vi "Load Machine Configuration.vi"(4 "error in (no error)":errorcluster, 6 "Reload?":bool, 7 "Instance Name":T2) -> (0 "error out":errorcluster, 3 "TC Parameters":T1)   [LabVIEW 2015, in "Config Data.lvlib" / "Config Data.lvclass"]
uses:
  Config Data.lvclass
  Startup Processes/_typedefs/Subpanel Names.ctl
  Startup Processes/Startup Processes.lvlib
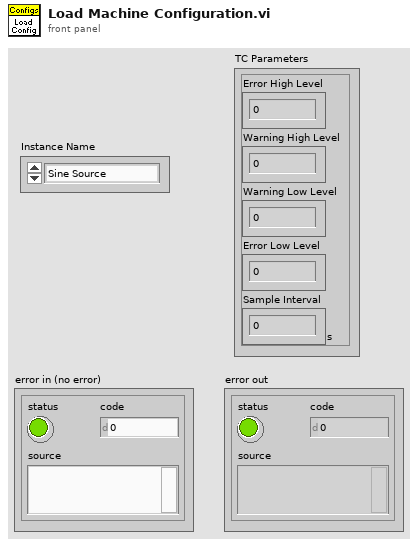
[diagram p1: front panel]
types:
  T1 = cluster{"Error High Level":dbl, "Warning High Level":dbl, "Warning Low Level":dbl, "Error Low Level":dbl, "Sample Interval":dbl[unit]}
  T2 = typedef "Startup Processes.lvlib/Subpanel Names.ctl" = enum16{"Sine Source", "Ramp Source", "Hen House TC", "Dog House TC", "Out House TC"}
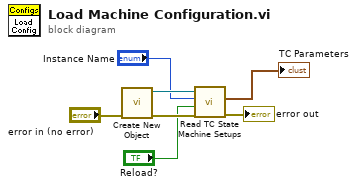
[diagram p0: block diagram]
diagram:
  n1 = call "Create New Object.vi"("Error In"="error in (no error)") -> ("Error Out"=w7:errorcluster, "Config Data"=w6:refnum<class "Config Data.lvclass">)  [unwired: 5 in]
  n2 = call-dynamic "Read TC State Machine Setups.vi"("Error In"=w7, "Reload?"="Reload?", "Instance Name"="Instance Name", "Config Data in"=w6) -> ("Error Out"=→"error out":errorcluster, "TC Parameters"=→"TC Parameters":T1)  [unwired: 1 in, 1 out]
